vi "Format PassFail Markdown List Item.vi"(8 "Error In":errorcluster, 11 "Pass/Fail Validation Input Cluster":T1) -> (0 "Error Out":errorcluster, 3 "Formatted Validation String List Item":string)   [LabVIEW 2017]
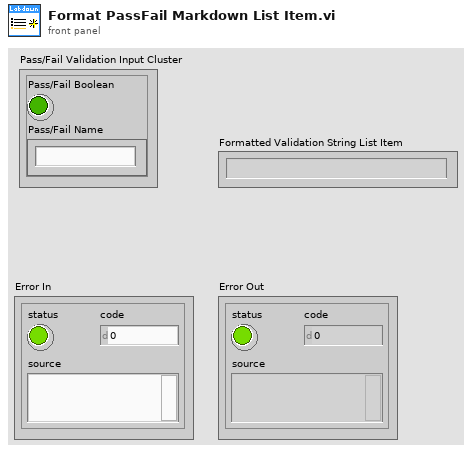
[diagram p1: front panel]
types:
  T1 = cluster{"Pass/Fail Boolean":bool, "Pass/Fail Name":string}
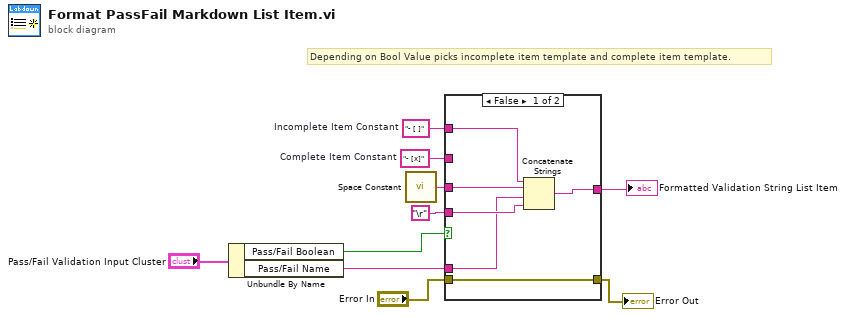
[diagram p0: block diagram]
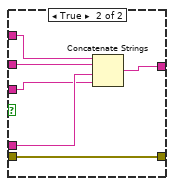
[diagram p2: hidden frame]
diagram:
  w6 = "- [x]"  # Complete Item Constant
  w5 = "- [ ]"  # Incomplete Item Constant
  # "Depending on Bool Value picks incomplete item template and complete item template."
  n1 = Unbundle By Name("Pass/Fail Validation Input Cluster") -> ("Pass/Fail Boolean"=w8:bool, "Pass/Fail Name"=w9:string)
  n2 = call <vilib>:"Space Constant.vi"() -> ("String"=w1:string)
  n3 = case shown="False" w8 {
    tunnel: w9 -> [w12 w19]
    tunnel: w6 -> [_ w22]
    tunnel: "\r" -> [w13 w17]
    tunnel: [w16 w21] -> w4
    tunnel: w5 -> [w15 _]
    tunnel: "Error In" -> [w14 w20]
    tunnel: [w14 w20] -> w2
    tunnel: w1 -> [w11 w18]
    frame False {
      n4 = Concatenate Strings(w15, w11, w12, w13) -> (w16:string)
    }
    frame True {
      n5 = Concatenate Strings(w22, w18, w19, w17) -> (w21:string)
    }
  }
  "Error Out" <- w2
  "Formatted Validation String List Item" <- w4
